vi "Resample(SubVI).vi"(1 "Divide by":i32=20, 2 "X":dbl[](array[numeric])) -> (0 "Y":dbl[](array[numeric]))   [LabVIEW 2017]
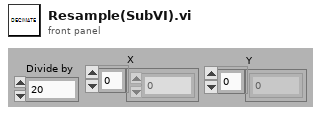
[diagram p1: front panel]
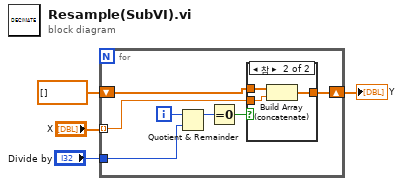
[diagram p0: block diagram]
diagram:
  n1 = for {
    tunnel: "X" -> [w9] mode=indexing
    shift-right: [w11] -> w1
    shift-left: dbl[] [] ("Y") -> [w10]
    tunnel: "Divide by" -> [w5]
    i -> [w7]
    n2 = Quotient & Remainder(x=w7, y=w5) -> (x-y*floor(x/y)=w8:i32)  [unwired: 1 out]
    n3 = Equal To 0?(x=w8) -> (x = 0?=w6:bool)
    n4 = case shown="참" w6 {
      tunnel: [w12 w15] -> w11
      tunnel: w10 -> [w12 w14]
      tunnel: w9 -> [_ w13]
      frame False {
      }
      frame True {
        n5 = Build Array (concatenate)(w14, w13) -> (w15:dbl[])
      }
    }
  }
  "Y" <- w1
